vi "Convert File Extension__ogtk.vi"   [LabVIEW 2018]
doc: "Converts the file extension of a file. \"new ending\" will accept an extension prefixed with or without a period, or a blank (\"\") string.\nFor example:\n\nfile name => c:\\temp\\data.txt\nnew ending => \"csv\" or \".csv\"\nnew filename => c:\\temp\\data.csv\nprev ending => \".txt\"\n\nfile name => c:\\temp\\data.txt\nnew ending => \"\"\nnew filename => c:\\temp\\data\nprev ending => \".txt\""
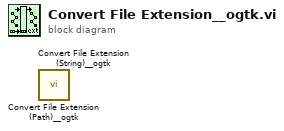
[diagram p0: block diagram]
diagram:
  n1 = call <userlib>:"Convert File Extension (Path)__ogtk.vi"() -> ()  [unwired: 2 in, 2 out]
  n2 = call <userlib>:"Convert File Extension (String)__ogtk.vi"() -> ()  [unwired: 2 in, 2 out]
